vi "Cycling_No_DAQ_Tasks_RT.vi"() -> ()   [LabVIEW 2020]
panel:
  out "PS Visa Out 3":refnum<visa-resource-name>
  out "PS error out 3":errorcluster
  in  "PS error in 3":errorcluster caption="PS error in (no error)"
  out "PS Visa Out 2":refnum<visa-resource-name>
  out "PS error out 2":errorcluster
  in  "PS error in 2":errorcluster caption="PS error in (no error)"
  out "PS error out":errorcluster
  out "PS Visa Out":refnum<visa-resource-name>
  in  "PS error in":errorcluster caption="PS error in (no error)"
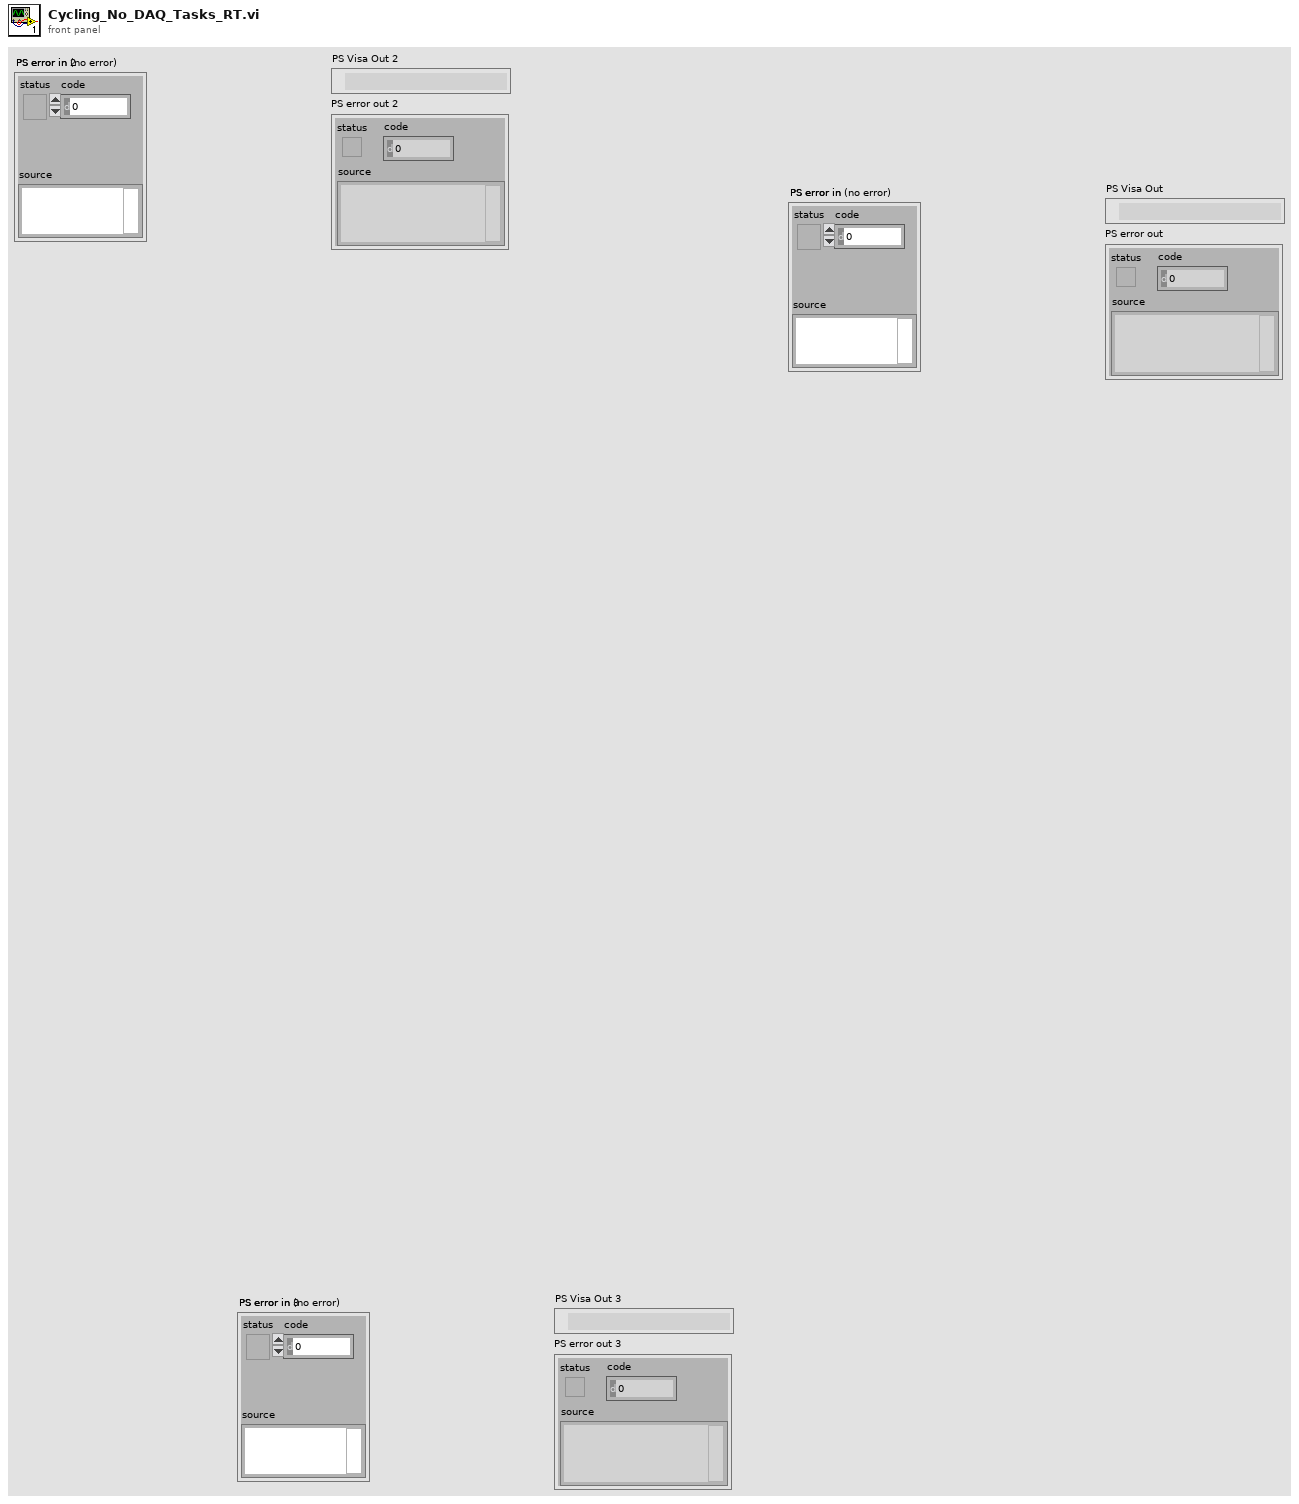
[diagram p1: front panel]
types:
  T1 = enum16{"\"30Q\"", "\"40T\"", "\"2P30Q\"", "\"3P30Q\"", "\"Nissan Leaf\""}
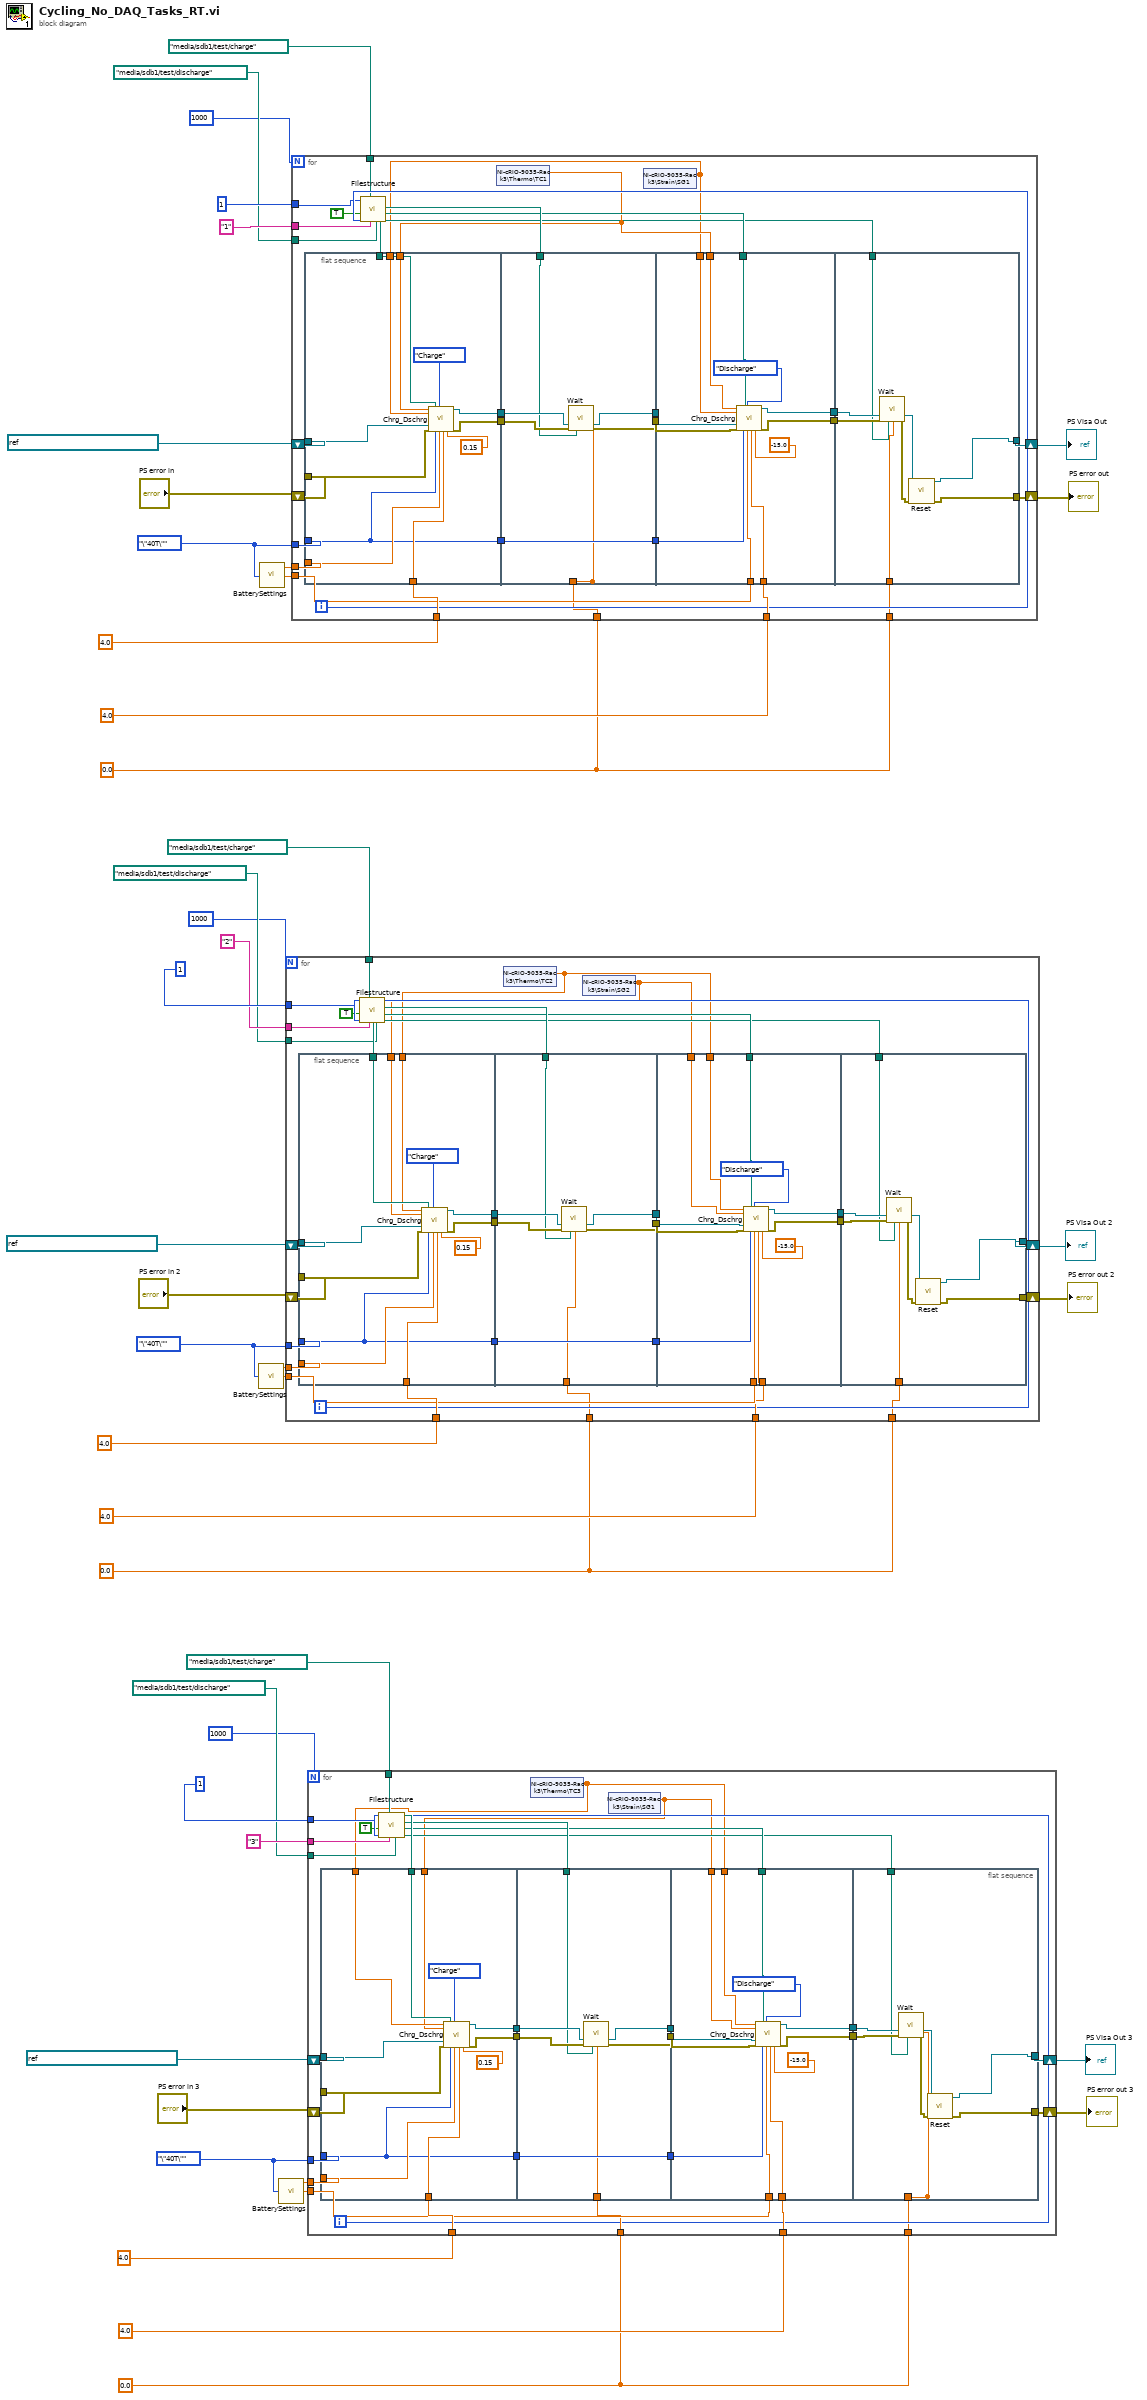
[diagram p0: block diagram]
diagram:
  w4 = T1."\"40T\"" ("Battery Type")
  w3 = 0.0 ("Wait time")
  w18 = T1."\"40T\"" ("Battery Type")
  w1 = 0.0 ("Wait time")
  w32 = T1."\"40T\"" ("Battery Type")
  w2 = 0.0 ("Wait time")
  n1 = call "BatterySettings.vi"("Battery Type"=w18) -> ("Min Voltage (V)"=w27:dbl, "Max Voltage (V)"=w29:dbl)  [unwired: 2 in, 1 out]
  n2 = call "BatterySettings.vi"("Battery Type"=w32) -> ("Min Voltage (V)"=w41:dbl, "Max Voltage (V)"=w43:dbl)  [unwired: 2 in, 1 out]
  n3 = call "BatterySettings.vi"("Battery Type"=w4) -> ("Min Voltage (V)"=w13:dbl, "Max Voltage (V)"=w15:dbl)  [unwired: 2 in, 1 out]
  n4 = for {
    N: 1000 ("Number of Cycles") -> [_]
    tunnel: w29 -> [w66]
    tunnel: w18 -> [w65]
    tunnel: 4.0 ("Charge Current Setpoint") -> [w64]
    tunnel: w27 -> [w63]
    tunnel: 4.0 ("Discharge Current Setpoint") -> [w62]
    shift-right: [w57] -> w24
    shift-left: refnum<visa-resource-name> "TCPIP0::192.168.0.202::inst0::INSTR" ("PS VISA in") -> [w68]
    shift-right: [w50] -> w25
    shift-left: "PS error in 2" -> [w67]
    tunnel: 1 ("Starting Cycle") -> [w55]
    tunnel: "2" ("Batteryname 2") -> [w53]
    tunnel: path "/media/sdb1/test/discharge" ("Discharge filepath") -> [w52]
    tunnel: path "/media/sdb1/test/charge" ("Charge filepath") -> [w51]
    tunnel: w1 -> [w49]
    tunnel: w1 -> [w48]
    i -> [w56]
    n5 = flat-sequence {
      tunnel: w68 -> [w79]
      tunnel: w67 -> [w80]
      tunnel: w65 -> [w81]
      tunnel: w66 -> [w82]
      tunnel: w64 -> [w83]
      tunnel: [w86] -> w76
      tunnel: [w85] -> w75
      tunnel: [w81] -> w74
      tunnel: w61 -> [w87]
      tunnel: w47 -> [w78]
      tunnel: w46 -> [w77]
      tunnel: w76 -> [w94]
      tunnel: w75 -> [w93]
      tunnel: [w89] -> w73
      tunnel: [w90] -> w72
      tunnel: w74 -> [w95]
      tunnel: [w95] -> w71
      tunnel: w60 -> [w92]
      tunnel: w48 -> [w91]
      tunnel: w73 -> [w102]
      tunnel: w72 -> [w103]
      tunnel: w71 -> [w104]
      tunnel: w63 -> [w105]
      tunnel: w62 -> [w106]
      tunnel: w59 -> [w101]
      tunnel: [w99] -> w70
      tunnel: [w98] -> w69
      tunnel: w47 -> [w97]
      tunnel: w46 -> [w96]
      tunnel: w58 -> [w110]
      tunnel: w70 -> [w115]
      tunnel: w69 -> [w114]
      tunnel: w49 -> [w111]
      tunnel: [w109] -> w57
      tunnel: [w108] -> w50
      frame #0 {
        n6 = call "Chrg_Dschrg.vi"("TC"=w78, "SG"=w77, "PS VISA in"=w79, "PS error in"=w80, "CyclePath"=w87, "Battery Type"=w81, "Charge/discharge"=enum8{"Charge", "Discharge"}."Charge", "Charge/Discharge Voltage Setpoint"=w82, "Current Setpoint"=w83, "Current Cutoff"=0.15) -> ("PS VISA out"=w86:refnum<visa-resource-name>, "PS error out"=w85:errorcluster)  [unwired: 6 in, 2 out]
      }
      frame #1 {
        n7 = call "Wait.vi"("PS VISA in"=w94, "PS error in"=w93, "Wait Filepath"=w92, "Wait time"=w91) -> ("PS Visa Out"=w89:refnum<visa-resource-name>, "PS error out"=w90:errorcluster)  [unwired: 10 in]
      }
      frame #2 {
        n8 = call "Chrg_Dschrg.vi"("TC"=w97, "SG"=w96, "PS VISA in"=w102, "PS error in"=w103, "CyclePath"=w101, "Battery Type"=w104, "Charge/discharge"=enum8{"Charge", "Discharge"}."Discharge", "Charge/Discharge Voltage Setpoint"=w105, "Current Setpoint"=w106, "Current Cutoff"=-15.0) -> ("PS VISA out"=w99:refnum<visa-resource-name>, "PS error out"=w98:errorcluster)  [unwired: 6 in, 2 out]
      }
      frame #3 {
        n9 = call "Wait.vi"("PS VISA in"=w115, "PS error in"=w114, "Wait Filepath"=w110, "Wait time"=w111) -> ("PS Visa Out"=w113:refnum<visa-resource-name>, "PS error out"=w112:errorcluster)  [unwired: 10 in]
        n10 = call "Reset.vi"("error in"=w112, "VISA resource name"=w113) -> ("error out"=w108:errorcluster, "VISA resource name out"=w109:refnum<visa-resource-name>)  [unwired: 8 in]
      }
    }
    n11 = call "Filestructure.vi"("Discharge filepath"=w52, "Batteryname"=w53, "Charge filepath"=w51, "For loop i"=w56, "In for loop"=TRUE, "Starting Cycle"=w55) -> ("DischargeWaitPath"=w58:path, "DischargeCyclePath"=w59:path, "ChargeWaitPath"=w60:path, "ChargeCyclePath"=w61:path)  [unwired: 1 in, 1 out]
    n12 = shared-variable "NI-cRIO-9035-Rack3\\Thermo\\TC2"() -> (w47:dbl)  [unwired: 1 in, 1 out]
    n13 = shared-variable "NI-cRIO-9035-Rack3\\Strain\\SG2"() -> (w46:dbl)  [unwired: 1 in, 1 out]
  }
  "PS error out 2" <- w25
  "PS Visa Out 2" <- w24
  n14 = for {
    N: 1000 ("Number of Cycles") -> [_]
    tunnel: w43 -> [w136]
    tunnel: w32 -> [w135]
    tunnel: 4.0 ("Charge Current Setpoint") -> [w134]
    tunnel: w41 -> [w133]
    tunnel: 4.0 ("Discharge Current Setpoint") -> [w132]
    tunnel: w2 -> [w118]
    shift-right: [w127] -> w38
    shift-left: refnum<visa-resource-name> "TCPIP0::192.168.0.201::inst0::INSTR" ("PS VISA in") -> [w138]
    shift-right: [w120] -> w39
    shift-left: "PS error in" -> [w137]
    tunnel: 1 ("Starting Cycle") -> [w125]
    tunnel: "1" ("Batteryname") -> [w123]
    tunnel: path "/media/sdb1/test/discharge" ("Discharge filepath") -> [w122]
    tunnel: path "/media/sdb1/test/charge" ("Charge filepath") -> [w121]
    tunnel: w2 -> [w119]
    i -> [w126]
    n15 = flat-sequence {
      tunnel: w138 -> [w149]
      tunnel: w137 -> [w150]
      tunnel: w135 -> [w151]
      tunnel: w136 -> [w152]
      tunnel: w134 -> [w153]
      tunnel: [w156] -> w146
      tunnel: [w155] -> w145
      tunnel: [w151] -> w144
      tunnel: w131 -> [w157]
      tunnel: w117 -> [w148]
      tunnel: w116 -> [w147]
      tunnel: w146 -> [w164]
      tunnel: w145 -> [w163]
      tunnel: [w160] -> w143
      tunnel: [w161] -> w142
      tunnel: w144 -> [w165]
      tunnel: [w165] -> w141
      tunnel: w130 -> [w162]
      tunnel: [w159] -> _
      tunnel: w118 -> [w159]
      tunnel: w143 -> [w172]
      tunnel: w142 -> [w173]
      tunnel: w141 -> [w174]
      tunnel: w133 -> [w175]
      tunnel: w132 -> [w176]
      tunnel: w129 -> [w171]
      tunnel: [w169] -> w140
      tunnel: [w168] -> w139
      tunnel: w117 -> [w167]
      tunnel: w116 -> [w166]
      tunnel: w128 -> [w180]
      tunnel: w140 -> [w185]
      tunnel: w139 -> [w184]
      tunnel: w119 -> [w181]
      tunnel: [w179] -> w127
      tunnel: [w178] -> w120
      frame #0 {
        n16 = call "Chrg_Dschrg.vi"("TC"=w148, "SG"=w147, "PS VISA in"=w149, "PS error in"=w150, "CyclePath"=w157, "Battery Type"=w151, "Charge/discharge"=enum8{"Charge", "Discharge"}."Charge", "Charge/Discharge Voltage Setpoint"=w152, "Current Setpoint"=w153, "Current Cutoff"=0.15) -> ("PS VISA out"=w156:refnum<visa-resource-name>, "PS error out"=w155:errorcluster)  [unwired: 6 in, 2 out]
      }
      frame #1 {
        n17 = call "Wait.vi"("PS VISA in"=w164, "PS error in"=w163, "Wait Filepath"=w162, "Wait time"=w159) -> ("PS Visa Out"=w160:refnum<visa-resource-name>, "PS error out"=w161:errorcluster)  [unwired: 10 in]
      }
      frame #2 {
        n18 = call "Chrg_Dschrg.vi"("TC"=w167, "SG"=w166, "PS VISA in"=w172, "PS error in"=w173, "CyclePath"=w171, "Battery Type"=w174, "Charge/discharge"=enum8{"Charge", "Discharge"}."Discharge", "Charge/Discharge Voltage Setpoint"=w175, "Current Setpoint"=w176, "Current Cutoff"=-15.0) -> ("PS VISA out"=w169:refnum<visa-resource-name>, "PS error out"=w168:errorcluster)  [unwired: 6 in, 2 out]
      }
      frame #3 {
        n19 = call "Wait.vi"("PS VISA in"=w185, "PS error in"=w184, "Wait Filepath"=w180, "Wait time"=w181) -> ("PS Visa Out"=w183:refnum<visa-resource-name>, "PS error out"=w182:errorcluster)  [unwired: 10 in]
        n20 = call "Reset.vi"("error in"=w182, "VISA resource name"=w183) -> ("error out"=w178:errorcluster, "VISA resource name out"=w179:refnum<visa-resource-name>)  [unwired: 8 in]
      }
    }
    n21 = call "Filestructure.vi"("Discharge filepath"=w122, "Batteryname"=w123, "Charge filepath"=w121, "For loop i"=w126, "In for loop"=TRUE, "Starting Cycle"=w125) -> ("DischargeWaitPath"=w128:path, "DischargeCyclePath"=w129:path, "ChargeWaitPath"=w130:path, "ChargeCyclePath"=w131:path)  [unwired: 1 in, 1 out]
    n22 = shared-variable "NI-cRIO-9035-Rack3\\Thermo\\TC1"() -> (w117:dbl)  [unwired: 1 in, 1 out]
    n23 = shared-variable "NI-cRIO-9035-Rack3\\Strain\\SG1"() -> (w116:dbl)  [unwired: 1 in, 1 out]
  }
  "PS error out" <- w39
  "PS Visa Out" <- w38
  n24 = for {
    N: 1000 ("Number of Cycles") -> [_]
    tunnel: w15 -> [w206]
    tunnel: w4 -> [w205]
    tunnel: 4.0 ("Charge Current Setpoint") -> [w204]
    tunnel: w13 -> [w203]
    tunnel: 4.0 ("Discharge Current Setpoint") -> [w202]
    tunnel: w3 -> [w197]
    shift-right: [w196] -> w10
    shift-left: refnum<visa-resource-name> "TCPIP0::192.168.0.204::inst0::INSTR" ("PS VISA in") -> [w208]
    shift-right: [w189] -> w11
    shift-left: "PS error in 3" -> [w207]
    tunnel: 1 ("Starting Cycle") -> [w194]
    tunnel: "3" ("Batteryname 3") -> [w192]
    tunnel: path "/media/sdb1/test/discharge" ("Discharge filepath") -> [w191]
    tunnel: path "/media/sdb1/test/charge" ("Charge filepath") -> [w190]
    tunnel: w3 -> [w188]
    i -> [w195]
    n25 = flat-sequence {
      tunnel: w208 -> [w219]
      tunnel: w207 -> [w220]
      tunnel: w205 -> [w221]
      tunnel: w206 -> [w222]
      tunnel: w204 -> [w223]
      tunnel: [w226] -> w216
      tunnel: [w225] -> w215
      tunnel: [w221] -> w214
      tunnel: w201 -> [w227]
      tunnel: w187 -> [w218]
      tunnel: w186 -> [w217]
      tunnel: w216 -> [w234]
      tunnel: w215 -> [w233]
      tunnel: [w229] -> w213
      tunnel: [w230] -> w212
      tunnel: w214 -> [w235]
      tunnel: [w235] -> w211
      tunnel: w200 -> [w232]
      tunnel: w197 -> [w231]
      tunnel: w213 -> [w242]
      tunnel: w212 -> [w243]
      tunnel: w211 -> [w244]
      tunnel: w203 -> [w245]
      tunnel: w202 -> [w246]
      tunnel: w199 -> [w241]
      tunnel: [w239] -> w210
      tunnel: [w238] -> w209
      tunnel: w187 -> [w237]
      tunnel: w186 -> [w236]
      tunnel: w198 -> [w251]
      tunnel: w210 -> [w255]
      tunnel: w209 -> [w254]
      tunnel: [w248] -> _
      tunnel: [w250] -> w196
      tunnel: [w249] -> w189
      tunnel: w188 -> [w248]
      frame #0 {
        n26 = call "Chrg_Dschrg.vi"("TC"=w218, "SG"=w217, "PS VISA in"=w219, "PS error in"=w220, "CyclePath"=w227, "Battery Type"=w221, "Charge/discharge"=enum8{"Charge", "Discharge"}."Charge", "Charge/Discharge Voltage Setpoint"=w222, "Current Setpoint"=w223, "Current Cutoff"=0.15) -> ("PS VISA out"=w226:refnum<visa-resource-name>, "PS error out"=w225:errorcluster)  [unwired: 6 in, 2 out]
      }
      frame #1 {
        n27 = call "Wait.vi"("PS VISA in"=w234, "PS error in"=w233, "Wait Filepath"=w232, "Wait time"=w231) -> ("PS Visa Out"=w229:refnum<visa-resource-name>, "PS error out"=w230:errorcluster)  [unwired: 10 in]
      }
      frame #2 {
        n28 = call "Chrg_Dschrg.vi"("TC"=w237, "SG"=w236, "PS VISA in"=w242, "PS error in"=w243, "CyclePath"=w241, "Battery Type"=w244, "Charge/discharge"=enum8{"Charge", "Discharge"}."Discharge", "Charge/Discharge Voltage Setpoint"=w245, "Current Setpoint"=w246, "Current Cutoff"=-15.0) -> ("PS VISA out"=w239:refnum<visa-resource-name>, "PS error out"=w238:errorcluster)  [unwired: 6 in, 2 out]
      }
      frame #3 {
        n29 = call "Wait.vi"("PS VISA in"=w255, "PS error in"=w254, "Wait Filepath"=w251, "Wait time"=w248) -> ("PS Visa Out"=w253:refnum<visa-resource-name>, "PS error out"=w252:errorcluster)  [unwired: 10 in]
        n30 = call "Reset.vi"("error in"=w252, "VISA resource name"=w253) -> ("error out"=w249:errorcluster, "VISA resource name out"=w250:refnum<visa-resource-name>)  [unwired: 8 in]
      }
    }
    n31 = call "Filestructure.vi"("Discharge filepath"=w191, "Batteryname"=w192, "Charge filepath"=w190, "For loop i"=w195, "In for loop"=TRUE, "Starting Cycle"=w194) -> ("DischargeWaitPath"=w198:path, "DischargeCyclePath"=w199:path, "ChargeWaitPath"=w200:path, "ChargeCyclePath"=w201:path)  [unwired: 1 in, 1 out]
    n32 = shared-variable "NI-cRIO-9035-Rack3\\Thermo\\TC3"() -> (w187:dbl)  [unwired: 1 in, 1 out]
    n33 = shared-variable "NI-cRIO-9035-Rack3\\Strain\\SG1"() -> (w186:dbl)  [unwired: 1 in, 1 out]
  }
  "PS error out 3" <- w11
  "PS Visa Out 3" <- w10
